vi "Configure Reporting Dialog.vi"(8 "error in (no error)":errorcluster, 11 "Execution UI In":refnum<class "Execution UI.lvclass">) -> (0 "error out":errorcluster, 2 "Reporting Enabled?":bool, 3 "Execution UI Out":refnum<class "Execution UI.lvclass">)   [LabVIEW 2020, in "Execution UI.lvclass"]
uses:
  Execution UI.lvclass
  Execution UI.lvclass/Execution UI.ctl
  Configuration Manager/Configuration Manager.lvclass
  Support/Utilities.lvlib
panel:
  in  "Open New Reports":bool
  in  "Report Path":path
  in  "Cancel":bool
  in  "Commit":bool
  in  "Reporting Enabled?":bool
  in  "Report Type":enum16{"Plain Text", "XML"}(ring)
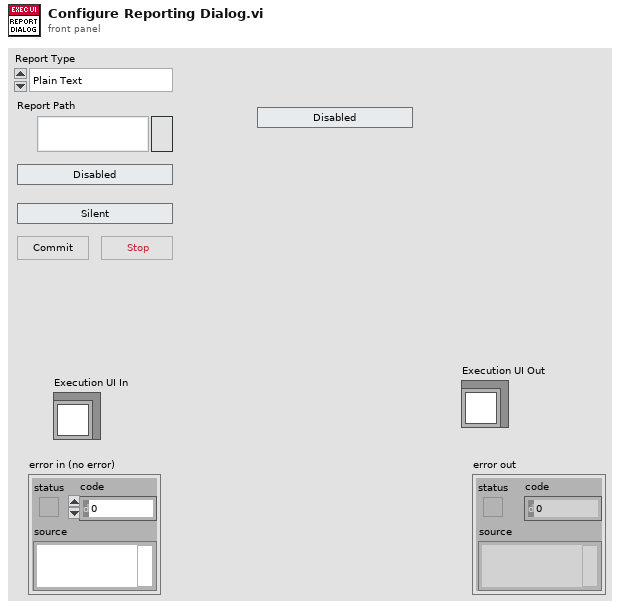
[diagram p1: front panel]
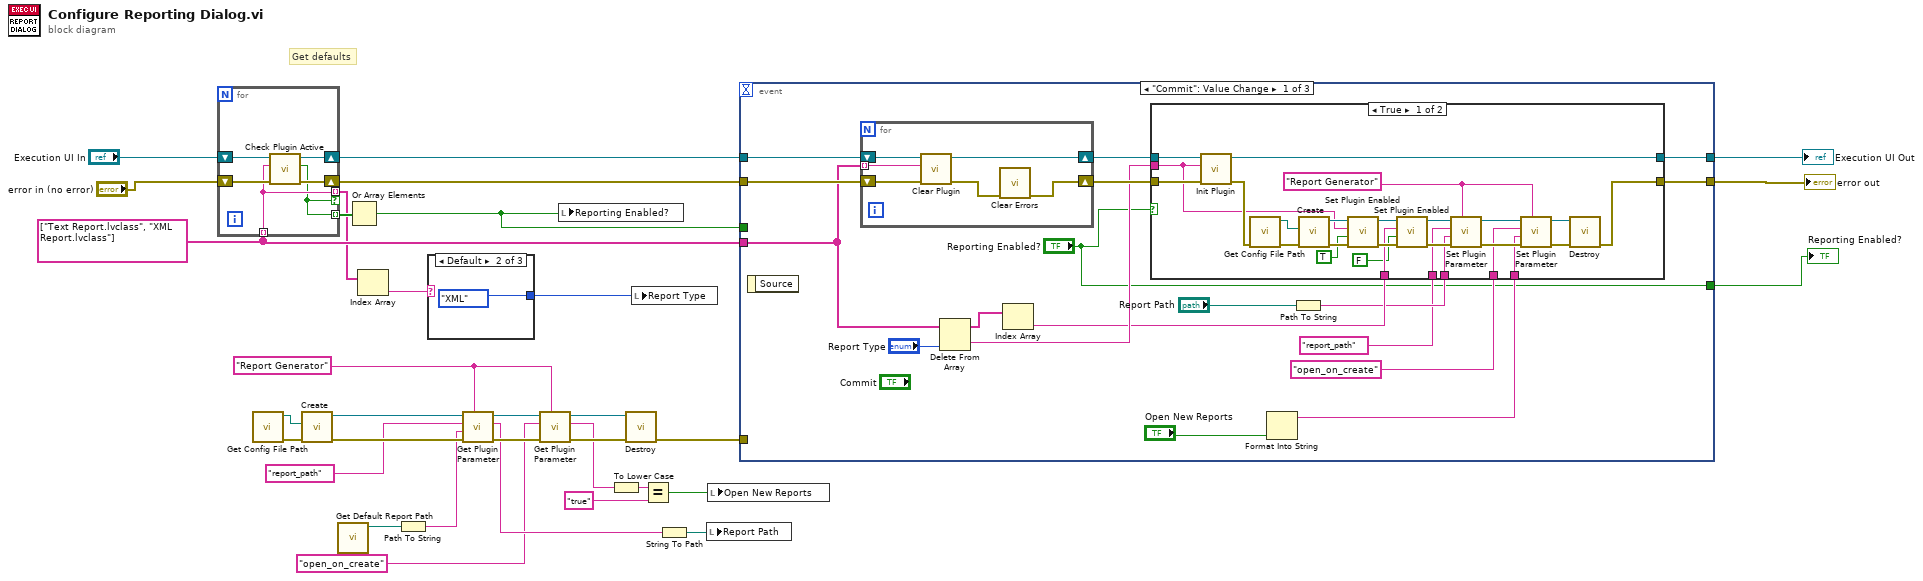
[diagram p0: block diagram]
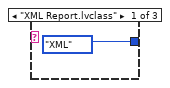
[diagram p2: hidden frame]
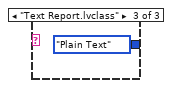
[diagram p3: hidden frame]
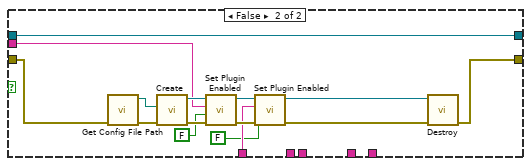
[diagram p4: hidden frame]
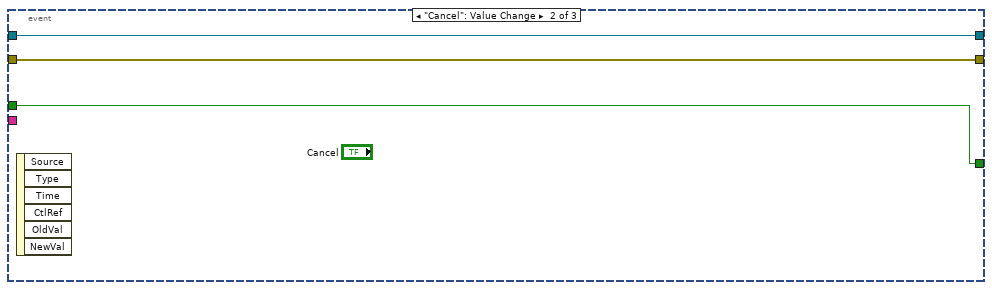
[diagram p5: hidden frame]
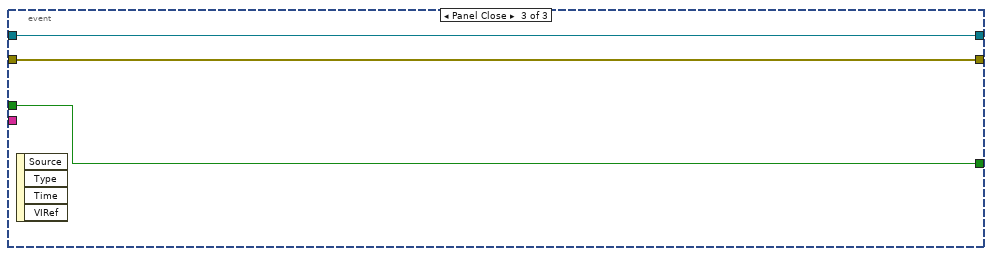
[diagram p6: hidden frame]
diagram:
  w1 = "Report Generator"
  w27 = string[] ["Text Report.lvclass", "XML Report.lvclass"] ("Plugin")
  # "Get defaults"
  n1 = for {
    shift-right: [w38] -> w30
    shift-left: "Execution UI In" -> [w39]
    shift-right: [w36] -> w28
    shift-left: "error in (no error)" -> [w37]
    tunnel: w27 -> [w35] mode=indexing
    tunnel: [w34] -> w26 mode=indexing
    tunnel: [w35] -> w21 mode=indexing if=w34
    n2 = call "Check Plugin Active.vi"("error in (no error)"=w37, "Plugin"=w35, "Execution UI in"=w39) -> ("error out"=w36:errorcluster, "Active?"=w34:bool, "Execution UI out"=w38:refnum<class "Execution UI.lvclass">)  [unwired: 6 in]
  }
  n3 = call "Get Config File Path.vi"() -> ("error out"=w24:errorcluster, "Config Directory"=w23:path)  [unwired: 10 in]
  n4 = call "Create.vi"("error in (no error)"=w24, "configuration file path"=w23) -> ("error out"=w18:errorcluster, "Configuration Manager out"=w25:refnum<class "Configuration Manager.lvclass">)  [unwired: 8 in]
  n5 = call "Get Default Report Path.vi"() -> ("Default Report Path"=w16:path)  [unwired: 10 in, 1 out]
  n6 = Or Array Elements(Boolean array=w26) -> (logical OR=w2:bool)
  n7 = Index Array(array=w21) -> (element=w19:string)  [unwired: 1 in]
  n8 = Path To String(path=w16) -> (string=w15:string)
  n9 = case shown="Default" w19 {
    tunnel: [enum16{"Plain Text", "XML"}."XML" ("f") enum16{"Plain Text", "XML"}."XML" ("f") enum16{"Plain Text", "XML"}."Plain Text" ("Report Type")] -> w20
    frame "XML Report.lvclass" {
    }
    frame Default {
    }
    frame "Text Report.lvclass" {
    }
  }
  n10 = call "Get Plugin Parameter.vi"("Plugin"=w1, "error in (no error)"=w18, "Default Value"=w15, "Name"="report_path", "Configuration Manager in"=w25) -> ("error out"=w22:errorcluster, "Value"=w13:string, "Configuration Manager out"=w11:refnum<class "Configuration Manager.lvclass">)  [unwired: 4 in]
  n11 = call "Get Plugin Parameter.vi"("Plugin"=w1, "error in (no error)"=w22, "Name"="open_on_create", "Configuration Manager in"=w11) -> ("error out"=w12:errorcluster, "Value"=w8:string, "Configuration Manager out"=w10:refnum<class "Configuration Manager.lvclass">)  [unwired: 5 in]
  n12 = local write "Reporting Enabled?"(w2) -> ()
  n13 = To Lower Case(string=w8) -> (all lower case string=w7:string)
  n14 = call "Destroy.vi"("error in (no error)"=w12, "Configuration Manager In"=w10) -> ("error out"=w4:errorcluster)  [unwired: 9 in]
  n15 = local write "Report Type"(w20) -> ()
  n16 = Equal?(x=w7, y="true") -> (x = y?=w5:bool)
  n17 = String To Path(string=w13) -> (path=w14:path)
  n18 = local write "Report Path"(w14) -> ()
  n19 = local write "Open New Reports"(w5) -> ()
  n20 = event shown="[0] \"Commit\": Value Change" {
    selector: _ -> [_ _ _]
    dyn-events: _ -> [_ _ _]
    timeout: _ -> [_ _ _]
    tunnel: [w55 w109 w112] -> w33
    tunnel: w30 -> [w60 w109 w112]
    tunnel: w28 -> [w59 w110 w113]
    tunnel: [w57 w110 w113] -> w32
    tunnel: w27 -> [w52 _ _]
    tunnel: w4 -> [_ _ _]
    tunnel: ["Reporting Enabled?" w108 w111] -> w3
    tunnel: w2 -> [_ w108 w111]
    event "Commit": Value Change {
      n21 = event-data() -> ()  [unwired: 1 in, 1 out]
      n22 = for {
        tunnel: w52 -> [w103] mode=indexing
        shift-right: [w107] -> w56
        shift-left: w60 -> [w106]
        shift-right: [w102] -> w58
        shift-left: w59 -> [w105]
        n23 = call "Clear Plugin.vi"("error in (no error)"=w105, "Plugin"=w103, "Execution UI in"=w106) -> ("error out"=w104:errorcluster, "Execution UI out"=w107:refnum<class "Execution UI.lvclass">)  [unwired: 7 in]
        n24 = call <vilib>:"Clear Errors.vi"("error in (no error)"=w104) -> ("error out"=w102:errorcluster)  [unwired: 5 in, 1 out]
      }
      n25 = Delete From Array(array=w52, index="Report Type") -> (deleted portion=w53:string, array with subset deleted=w51:string[])  [unwired: 1 in]
      n26 = Index Array(array=w51) -> (element=w50:string)  [unwired: 1 in]
      n27 = Format Into String("Open New Reports") -> (resulting string=w44:string)  [unwired: 3 in, 1 out]
      n28 = Path To String(path="Report Path") -> (string=w48:string)
      n29 = case shown="True" "Reporting Enabled?" {
        tunnel: w58 -> [w86 w101]
        tunnel: [w78 w95] -> w57
        tunnel: w56 -> [w85 w100]
        tunnel: [w84 w100] -> w55
        tunnel: w53 -> [w69 w94]
        tunnel: w50 -> [w74 w89]
        tunnel: w48 -> [w68 _]
        tunnel: "report_path" ("Name") -> [w67 _]
        tunnel: "open_on_create" ("Name") -> [w63 _]
        tunnel: w44 -> [w62 _]
        frame True {
          w61 = "Report Generator"
          n30 = call "Init Plugin.vi"("error in (no error)"=w86, "Plugin"=w69, "Execution UI in"=w85) -> ("error out"=w79:errorcluster, "Execution UI out"=w84:refnum<class "Execution UI.lvclass">)  [unwired: 7 in]
          n31 = call "Get Config File Path.vi"("error in (no error)"=w79) -> ("error out"=w80:errorcluster, "Config Directory"=w72:path)  [unwired: 9 in]
          n32 = call "Create.vi"("error in (no error)"=w80, "configuration file path"=w72) -> ("error out"=w82:errorcluster, "Configuration Manager out"=w81:refnum<class "Configuration Manager.lvclass">)  [unwired: 8 in]
          n33 = call "Set Plugin Enabled.vi"("error in (no error)"=w82, "Enabled?"=TRUE, "Plugin"=w69, "Configuration Manager in"=w81) -> ("error out"=w83:errorcluster, "Configuration Manager out"=w75:refnum<class "Configuration Manager.lvclass">)  [unwired: 6 in]
          n34 = call "Set Plugin Enabled.vi"("error in (no error)"=w83, "Enabled?"=FALSE, "Plugin"=w74, "Configuration Manager in"=w75) -> ("error out"=w76:errorcluster, "Configuration Manager out"=w70:refnum<class "Configuration Manager.lvclass">)  [unwired: 6 in]
          n35 = call "Set Plugin Parameter.vi"("Plugin"=w61, "error in (no error)"=w76, "Value"=w68, "Name"=w67, "Configuration Manager in"=w70) -> ("error out"=w71:errorcluster, "Configuration Manager out"=w65:refnum<class "Configuration Manager.lvclass">)  [unwired: 5 in]
          n36 = call "Set Plugin Parameter.vi"("Plugin"=w61, "error in (no error)"=w71, "Value"=w62, "Name"=w63, "Configuration Manager in"=w65) -> ("error out"=w66:errorcluster, "Configuration Manager out"=w64:refnum<class "Configuration Manager.lvclass">)  [unwired: 5 in]
          n37 = call "Destroy.vi"("error in (no error)"=w66, "Configuration Manager In"=w64) -> ("error out"=w78:errorcluster)  [unwired: 9 in]
        }
        frame False {
          n38 = call "Get Config File Path.vi"("error in (no error)"=w101) -> ("error out"=w96:errorcluster, "Config Directory"=w87:path)  [unwired: 9 in]
          n39 = call "Create.vi"("error in (no error)"=w96, "configuration file path"=w87) -> ("error out"=w98:errorcluster, "Configuration Manager out"=w97:refnum<class "Configuration Manager.lvclass">)  [unwired: 8 in]
          n40 = call "Set Plugin Enabled.vi"("error in (no error)"=w98, "Enabled?"=FALSE, "Plugin"=w94, "Configuration Manager in"=w97) -> ("error out"=w99:errorcluster, "Configuration Manager out"=w91:refnum<class "Configuration Manager.lvclass">)  [unwired: 6 in]
          n41 = call "Set Plugin Enabled.vi"("error in (no error)"=w99, "Enabled?"=FALSE, "Plugin"=w89, "Configuration Manager in"=w91) -> ("error out"=w92:errorcluster, "Configuration Manager out"=w90:refnum<class "Configuration Manager.lvclass">)  [unwired: 6 in]
          n42 = call "Destroy.vi"("error in (no error)"=w92, "Configuration Manager In"=w90) -> ("error out"=w95:errorcluster)  [unwired: 9 in]
        }
      }
    }
    event "Cancel": Value Change {
      n43 = event-data() -> ()  [unwired: 1 in, 6 out]
    }
    event Panel Close {
      n44 = event-data() -> ()  [unwired: 1 in, 4 out]
    }
  }
  "error out" <- w32
  "Execution UI Out" <- w33
  "Reporting Enabled?" <- w3
